vi "SignalConversion.vi"(1 "Method for Zbead calculation (hard coded)":u16(ring) items=["Linear", "Polynomial", "Lookup table"], 6 "Reinitialize time? (F)":bool, 8 "error in (no error)":errorcluster, 9 "All data after scaling":T2, 10 "All DAQ channels":T1, 11 "Params in":T8={"Manual Control"={"Rotation Control"={"Phase"=0.0, "A amp (0-120)"=75.0, "B amp (0-120)"=53.3, "mean freq  [MHz]\ndefault 39.99"=40.0, "freq difference [Hz]"=2.0, "Enable A"=TRUE, "Enable B"=TRUE}, "X piezo\n [nm]"=0.0, "Y peizo\n [nm]"=0.0, "-Z piezo\n [nm]"=5.012658227848101, "AOM0 \nPower"=0.2}, "Piezo Calibr"={"Px2Vx(AO)"=nan, "Py2Vy(AO)"=nan, "Pz2Vz(AO)"=nan, "Min Px"=nan, "Min Py"=nan, "Min Pz"=nan, "Max Px"=nan, "Max Py"=nan, "Max Pz"=nan, "Vx0 (V)"=nan, "Vy0 (V)"=nan, "Vz0 (V)"=nan}, "Instrument Calibr"={"Angular compensation coeffs"=[], "TetherCenter"={"TrapX_AO 0 [nm]"=nan, "TrapY_AO 0 [nm]"=nan, "TrapZ_AO 0 [nm]"=nan}, "XYZsignal baseline"={"Xsignal0"=nan, "Ysignal0"=nan, "Zsignal0"=nan, "Zsig slope"=nan, "Z bead0"=nan}, "S and P to Vs0"={"Vs0/P"=1.0, "Vs0/S"=1.0}, "Psi"=0.0, "ePS:eRL drift correlation"={"Interc P"=nan, "Slope P"=nan, "Interc S"=nan, "Slope S"=nan}, "Current piezo volt AO"={"Vpx_AO [V]"=nan, "Vpy_AO [V]"=nan, "Vpz_AO [V]"=nan}}, "Cylinder Calibr"={"ZStiff"=nan, "Zsens"=nan, "AngStiff"=nan, "XStiff"=nan, "Xsens"=nan, "MaxEllip"=nan, "YStiff"=nan, "Ysens"=nan, "FocalShift"=nan, "Sfz"=nan, "1/Sz"=nan, "Stau"=nan, "Sfx"=nan, "1/Sx"=nan, "1/Sang"=nan, "Sfy"=nan, "1/Sy"=nan, "1/focal"=nan}, "DAQParams"={"Buffer size"=nan, "Scanning rate"=nan, "Average"=nan, "Sampling rate"=nan, "set dt"=nan}, "DAQ channel offsets"={"A0 [V]"=0.0, "D0 [V]"=0.0, "P0  [V]"=0.0, "S0 [V]"=0.0, "L0 [V]"=0.0, "R0 [V]"=0.0, "Vpx0 [V]"=0.0, "Vpy0 [V]"=0.0, "Vpz0 [V]"=0.0, "Vsum0 [V]"=0.0, "Vpx_AO0 [V]"=0.0, "Vpy_AO0 [V]"=0.0, "Vpz_AO0 [V]"=0.0}, "Z bead polynomial coeffs"=[nan, nan, nan, nan], "Skip button ref"=refnum, "z bead lookup table"={"z signal"=[], "z bead"=[]}, "SP->power Matrix"=[], "Ms2p"=[], "Mp2s"=[], "Polynomial coeff V_px,y,z 2 position (nm)"=[], "task in"=""} {"Instrument Calibr"."Psi" format="%#_2f"; "Manual Control"."Y peizo\n [nm]" scale=0.0..7000.0; "Manual Control"."AOM0 \nPower" scale=0.0..1.0; "Manual Control"."X piezo\n [nm]" scale=0.0..7000.0; "Manual Control"."Rotation Control"."freq difference [Hz]" step=0.5; "Manual Control"."Rotation Control"."mean freq  [MHz]\ndefault 39.99" min=0.0 step=0.01; "Manual Control"."Rotation Control"."B amp (0-120)" min=0.0 max=120.0 step=0.1; "Manual Control"."Rotation Control"."A amp (0-120)" min=0.0 max=120.0 step=0.1; "Manual Control"."Rotation Control"."Phase" scale=0.0..360.0; "Manual Control"."-Z piezo\n [nm]" scale=1000.0..7000.0}) -> (0 "error out":errorcluster, 2 "Physical Quantities cluster out":T13, 3 "Params out":T8={"Manual Control"={"Rotation Control"={"Phase"=0.0, "A amp (0-120)"=75.0, "B amp (0-120)"=53.3, "mean freq  [MHz]\ndefault 39.99"=40.0, "freq difference [Hz]"=2.0, "Enable A"=TRUE, "Enable B"=TRUE}, "X piezo\n [nm]"=0.0, "Y peizo\n [nm]"=0.0, "-Z piezo\n [nm]"=5.012658227848101, "AOM0 \nPower"=0.2}, "Piezo Calibr"={"Px2Vx(AO)"=nan, "Py2Vy(AO)"=nan, "Pz2Vz(AO)"=nan, "Min Px"=nan, "Min Py"=nan, "Min Pz"=nan, "Max Px"=nan, "Max Py"=nan, "Max Pz"=nan, "Vx0 (V)"=nan, "Vy0 (V)"=nan, "Vz0 (V)"=nan}, "Instrument Calibr"={"Angular compensation coeffs"=[], "TetherCenter"={"TrapX_AO 0 [nm]"=nan, "TrapY_AO 0 [nm]"=nan, "TrapZ_AO 0 [nm]"=nan}, "XYZsignal baseline"={"Xsignal0"=nan, "Ysignal0"=nan, "Zsignal0"=nan, "Zsig slope"=nan, "Z bead0"=nan}, "S and P to Vs0"={"Vs0/P"=1.0, "Vs0/S"=1.0}, "Psi"=0.0, "ePS:eRL drift correlation"={"Interc P"=nan, "Slope P"=nan, "Interc S"=nan, "Slope S"=nan}, "Current piezo volt AO"={"Vpx_AO [V]"=nan, "Vpy_AO [V]"=nan, "Vpz_AO [V]"=nan}}, "Cylinder Calibr"={"ZStiff"=nan, "Zsens"=nan, "AngStiff"=nan, "XStiff"=nan, "Xsens"=nan, "MaxEllip"=nan, "YStiff"=nan, "Ysens"=nan, "FocalShift"=nan, "Sfz"=nan, "1/Sz"=nan, "Stau"=nan, "Sfx"=nan, "1/Sx"=nan, "1/Sang"=nan, "Sfy"=nan, "1/Sy"=nan, "1/focal"=nan}, "DAQParams"={"Buffer size"=nan, "Scanning rate"=nan, "Average"=nan, "Sampling rate"=nan, "set dt"=nan}, "DAQ channel offsets"={"A0 [V]"=0.0, "D0 [V]"=0.0, "P0  [V]"=0.0, "S0 [V]"=0.0, "L0 [V]"=0.0, "R0 [V]"=0.0, "Vpx0 [V]"=0.0, "Vpy0 [V]"=0.0, "Vpz0 [V]"=0.0, "Vsum0 [V]"=0.0, "Vpx_AO0 [V]"=0.0, "Vpy_AO0 [V]"=0.0, "Vpz_AO0 [V]"=0.0}, "Z bead polynomial coeffs"=[nan, nan, nan, nan], "Skip button ref"=refnum, "z bead lookup table"={"z signal"=[], "z bead"=[]}, "SP->power Matrix"=[], "Ms2p"=[], "Mp2s"=[], "Polynomial coeff V_px,y,z 2 position (nm)"=[], "task in"=""} {"Instrument Calibr"."Psi" format="%#_2f"; "Manual Control"."Y peizo\n [nm]" scale=0.0..7000.0; "Manual Control"."AOM0 \nPower" scale=0.0..1.0; "Manual Control"."X piezo\n [nm]" scale=0.0..7000.0; "Manual Control"."Rotation Control"."freq difference [Hz]" step=0.5; "Manual Control"."Rotation Control"."mean freq  [MHz]\ndefault 39.99" min=0.0 step=0.01; "Manual Control"."Rotation Control"."B amp (0-120)" min=0.0 max=120.0 step=0.1; "Manual Control"."Rotation Control"."A amp (0-120)" min=0.0 max=120.0 step=0.1; "Manual Control"."Rotation Control"."Phase" scale=0.0..360.0; "Manual Control"."-Z piezo\n [nm]" scale=1000.0..7000.0})   [LabVIEW 2017, in "SignalConverson.lvlib"]
uses:
  SignalConverson.lvlib
  Initialization/New Param_170907.ctl
  Initialization/ManualCtrl.ctl
  Initialization/CylinderCalibrNew.ctl
  DAQChannelOffsets.ctl
  <vilib>/Analysis/Matrix/Datatypes/RealMatrix.ctl
  Initialization/Physical Quantitites.ctl
  ScaledData.ctl
  Measrured TrapXYZ.ctl
  Data Before Angle Compensation.ctl
  Angle compensated data.ctl
  XYZ Signals.ctl
  Set TrapXYZ.ctl
  DAQChannelRawData.ctl
  <vilib>/Analysis/polynomials.llb/Scalar Polynomial Evaluation (DBL).vi
  <vilib>/Analysis/NI_AALPro.lvlib
  Initialization/Initialization.lvlib
  <vilib>/Analysis/Matrix/NI_Matrix.lvlib
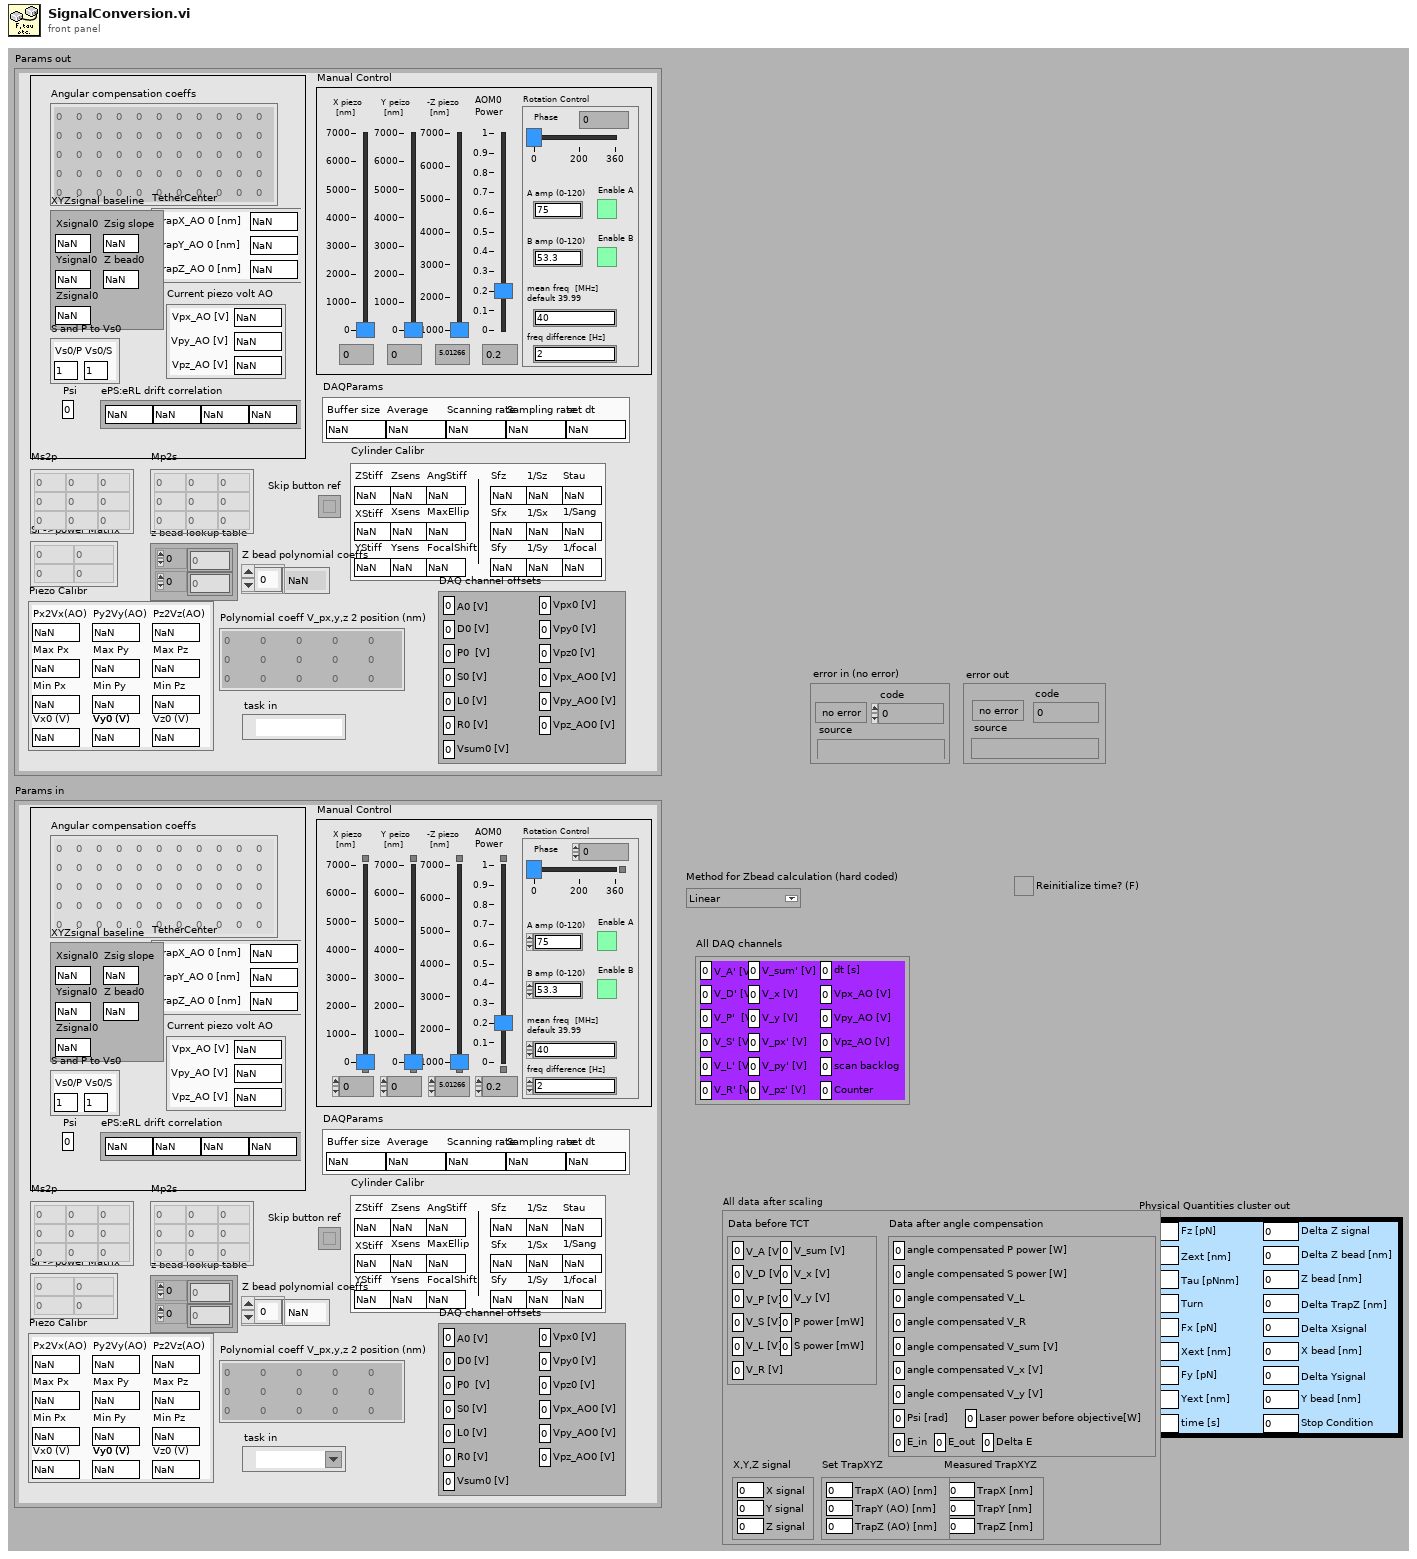
[diagram p1: front panel]
types:
  T1 = typedef "SignalConverson.lvlib/DAQChannelRawData.ctl" = cluster{"V_A' [V]":dbl, "V_D' [V]":dbl, "V_P'  [V]":dbl, "V_S' [V]":dbl, "V_L' [V]":dbl, "V_R' [V]":dbl, "V_sum' [V]":dbl, "V_x [V]":dbl, "V_y [V]":dbl, "V_px' [V]":dbl, "V_py' [V]":dbl, "V_pz' [V]":dbl, "dt [s]":dbl, "Vpx_AO [V]":dbl, "Vpy_AO [V]":dbl, "Vpz_AO [V]":dbl, "scan backlog":u32, "Counter":u32}
  T2 = typedef "SignalConverson.lvlib/ScaledData.ctl" = cluster{"Measured TrapXYZ":T3, "Data before TCT":T4, "Data after angle compensation":T5, "X,Y,Z signal":T6, "Set TrapXYZ":T7}
  T3 = typedef "SignalConverson.lvlib/Measrured TrapXYZ.ctl" = cluster{"TrapX [nm]":dbl, "TrapY [nm]":dbl, "TrapZ [nm]":dbl}
  T4 = typedef "SignalConverson.lvlib/Data Before Angle Compensation.ctl" = cluster{"V_A [V]":dbl, "V_D [V]":dbl, "V_P [V]":dbl, "V_S [V]":dbl, "V_L [V]":dbl, "V_R [V]":dbl, "V_sum [V]":dbl, "V_x [V]":dbl, "V_y [V]":dbl, "P power [mW]":dbl, "S power [mW]":dbl}
  T5 = typedef "SignalConverson.lvlib/Angle compensated data.ctl" = cluster{"angle compensated P power [W]":dbl, "angle compensated S power [W]":dbl, "angle compensated V_L":dbl, "angle compensated V_R":dbl, "angle compensated V_sum [V]":dbl, "angle compensated V_x [V]":dbl, "angle compensated V_y [V]":dbl, "Psi [rad]":dbl, "Laser power before objective[W]":dbl, "E_in":dbl, "E_out":dbl, "Delta E":dbl}
  T6 = typedef "SignalConverson.lvlib/XYZ Signals.ctl" = cluster{"X signal":dbl, "Y signal":dbl, "Z signal":dbl}
  T7 = typedef "SignalConverson.lvlib/Set TrapXYZ.ctl" = cluster{"TrapX (AO) [nm]":dbl, "TrapY (AO) [nm]":dbl, "TrapZ (AO) [nm]":dbl}
  T8 = typedef "Initialization.lvlib/New Param_170907.ctl" = cluster{"Manual Control":T9, "Piezo Calibr":cluster{"Px2Vx(AO)":dbl, "Py2Vy(AO)":dbl, "Pz2Vz(AO)":dbl, "Min Px":dbl, "Min Py":dbl, "Min Pz":dbl, "Max Px":dbl, "Max Py":dbl, "Max Pz":dbl, "Vx0 (V)":dbl, "Vy0 (V)":dbl, "Vz0 (V)":dbl}, "Instrument Calibr":cluster{"Angular compensation coeffs":dbl[][], "TetherCenter":cluster{"TrapX_AO 0 [nm]":dbl, "TrapY_AO 0 [nm]":dbl, "TrapZ_AO 0 [nm]":dbl}, "XYZsignal baseline":cluster{"Xsignal0":dbl, "Ysignal0":dbl, "Zsignal0":dbl, "Zsig slope":dbl, "Z bead0":dbl}, "S and P to Vs0":cluster{"Vs0/P":dbl, "Vs0/S":dbl}, "Psi":dbl, "ePS:eRL drift correlation":cluster{"Interc P":dbl, "Slope P":dbl, "Interc S":dbl, "Slope S":dbl}, "Current piezo volt AO":cluster{"Vpx_AO [V]":dbl, "Vpy_AO [V]":dbl, "Vpz_AO [V]":dbl}}, "Cylinder Calibr":T10, "DAQParams":cluster{"Buffer size":dbl, "Scanning rate":dbl, "Average":dbl, "Sampling rate":dbl, "set dt":dbl}, "DAQ channel offsets":T11, "Z bead polynomial coeffs":dbl[], "Skip button ref":refnum<vi>, "z bead lookup table":cluster{"z signal":dbl[], "z bead":dbl[]}, "SP->power Matrix":T12, "Ms2p":T12, "Mp2s":T12, "Polynomial coeff V_px,y,z 2 position (nm)":dbl[][], "task in":refnum<k21>}
  T9 = typedef "Initialization.lvlib/ManualCtrl.ctl" = cluster{"Rotation Control":cluster{"Phase":dbl, "A amp (0-120)":dbl, "B amp (0-120)":dbl, "mean freq  [MHz]\ndefault 39.99":dbl, "freq difference [Hz]":dbl, "Enable A":bool, "Enable B":bool}, "X piezo\n [nm]":dbl, "Y peizo\n [nm]":dbl, "-Z piezo\n [nm]":dbl, "AOM0 \nPower":dbl}
  T10 = typedef "Initialization.lvlib/CylinderCalibrNew.ctl" = cluster{"ZStiff":dbl, "Zsens":dbl, "AngStiff":dbl, "XStiff":dbl, "Xsens":dbl, "MaxEllip":dbl, "YStiff":dbl, "Ysens":dbl, "FocalShift":dbl, "Sfz":dbl, "1/Sz":dbl, "Stau":dbl, "Sfx":dbl, "1/Sx":dbl, "1/Sang":dbl, "Sfy":dbl, "1/Sy":dbl, "1/focal":dbl}
  T11 = typedef "SignalConverson.lvlib/DAQChannelOffsets.ctl" = cluster{"A0 [V]":dbl, "D0 [V]":dbl, "P0  [V]":dbl, "S0 [V]":dbl, "L0 [V]":dbl, "R0 [V]":dbl, "Vpx0 [V]":dbl, "Vpy0 [V]":dbl, "Vpz0 [V]":dbl, "Vsum0 [V]":dbl, "Vpx_AO0 [V]":dbl, "Vpy_AO0 [V]":dbl, "Vpz_AO0 [V]":dbl}
  T12 = typedef "NI_Matrix.lvlib/RealMatrix.ctl" = dbl[][]
  T13 = typedef "SignalConverson.lvlib/Physical Quantitites.ctl" = cluster{"Fz [pN]":dbl, "Zext [nm]":dbl, "Tau [pNnm]":dbl, "Turn":dbl, "Fx [pN]":dbl, "Xext [nm]":dbl, "Fy [pN]":dbl, "Yext [nm]":dbl, "time [s]":dbl, "Delta Z signal":dbl, "Delta Z bead [nm]":dbl, "Z bead [nm]":dbl, "Delta TrapZ [nm]":dbl, "Delta Xsignal":dbl, "X bead [nm]":dbl, "Delta Ysignal":dbl, "Y bead [nm]":dbl, "Stop Condition":dbl}
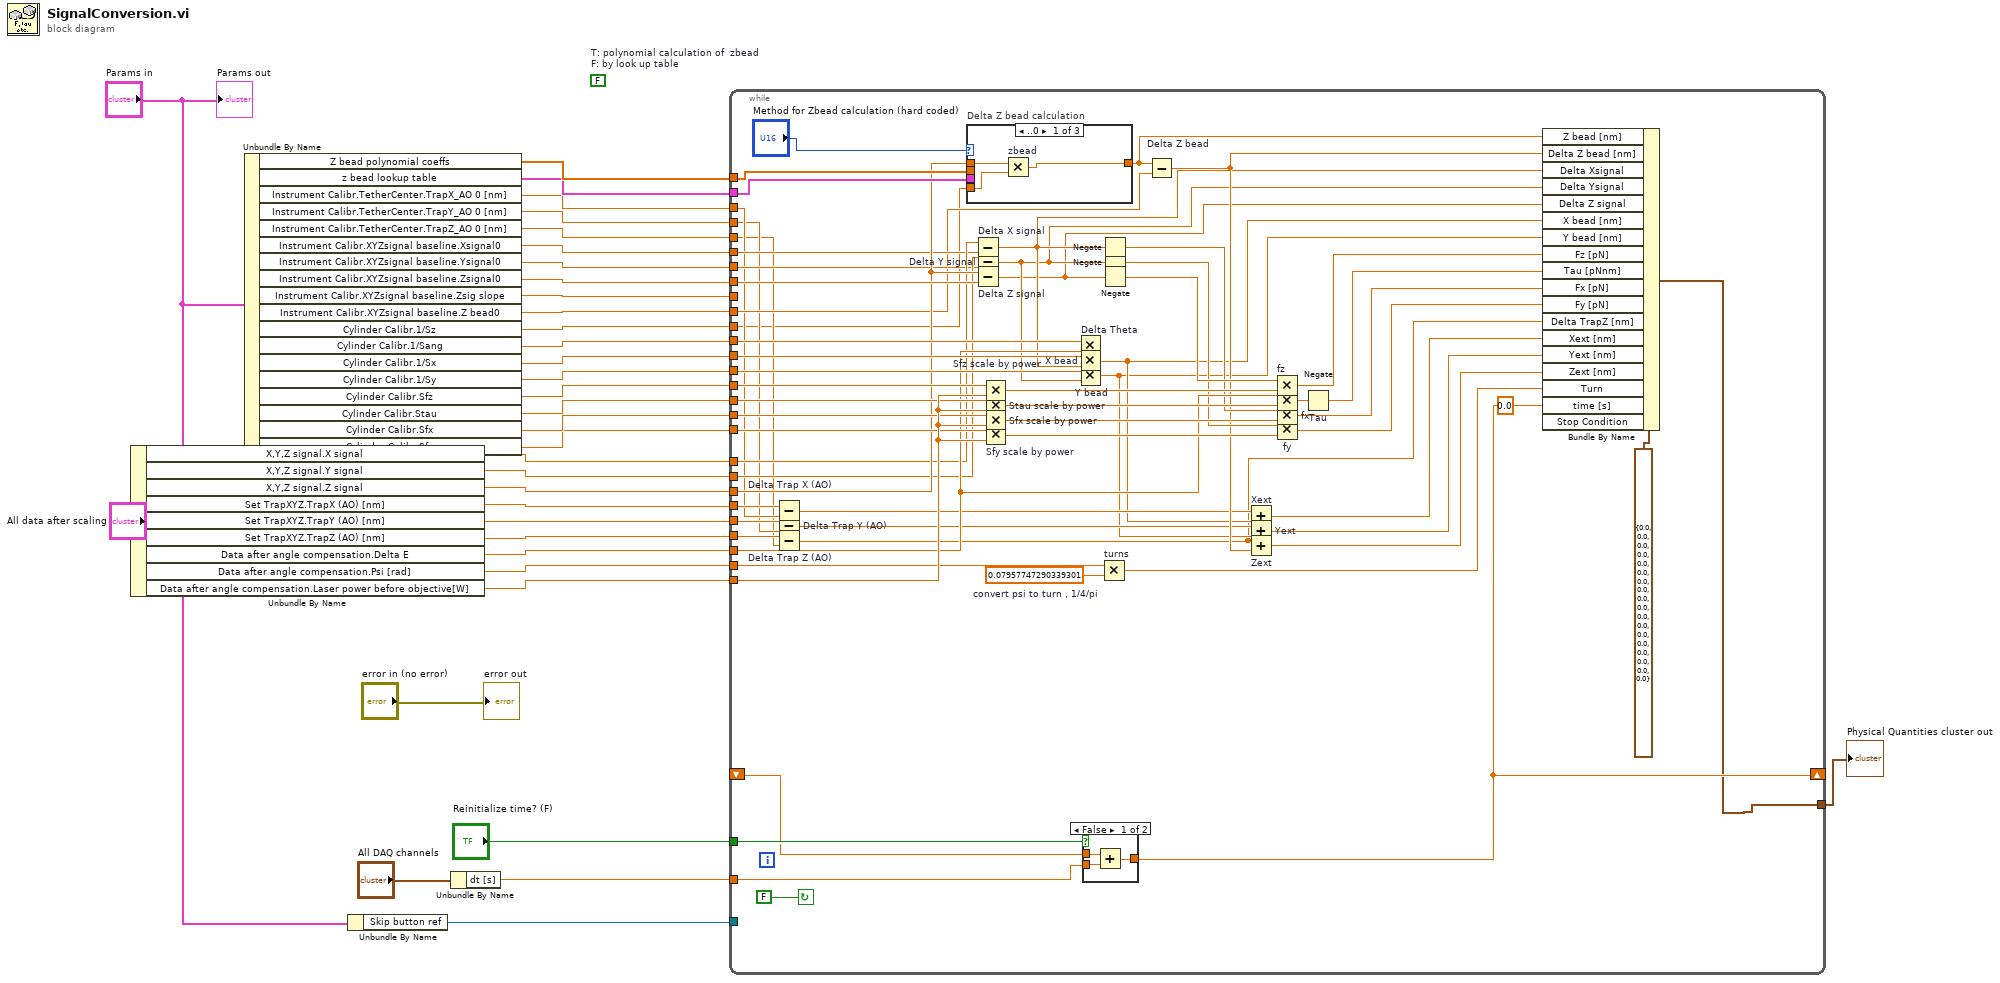
[diagram p0: block diagram]
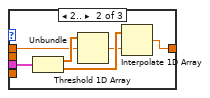
[diagram p2: hidden frame]
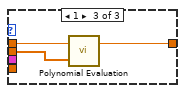
[diagram p3: hidden frame]
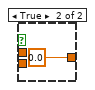
[diagram p4: hidden frame]
diagram:
  (unwired) FALSE  # T: polynomial calculation of  zbead F: by look up table
  n1 = Unbundle By Name("All data after scaling") -> ("X,Y,Z signal.X signal"=w29:dbl, "X,Y,Z signal.Y signal"=w30:dbl, "X,Y,Z signal.Z signal"=w31:dbl, "Set TrapXYZ.TrapX (AO) [nm]"=w28:dbl, "Set TrapXYZ.TrapY (AO) [nm]"=w27:dbl, "Set TrapXYZ.TrapZ (AO) [nm]"=w26:dbl, "Data after angle compensation.Delta E"=w25:dbl, "Data after angle compensation.Psi [rad]"=w24:dbl, "Data after angle compensation.Laser power before objective[W]"=w21:dbl)
  n2 = Unbundle By Name("Params in") -> ("Z bead polynomial coeffs"=w34:dbl[], "z bead lookup table"=w33:cluster{"z signal":dbl[], "z bead":dbl[]}, "Instrument Calibr.TetherCenter.TrapX_AO 0 [nm]"=w20:dbl, "Instrument Calibr.TetherCenter.TrapY_AO 0 [nm]"=w19:dbl, "Instrument Calibr.TetherCenter.TrapZ_AO 0 [nm]"=w18:dbl, "Instrument Calibr.XYZsignal baseline.Xsignal0"=w17:dbl, "Instrument Calibr.XYZsignal baseline.Ysignal0"=w16:dbl, "Instrument Calibr.XYZsignal baseline.Zsignal0"=w15:dbl, "Instrument Calibr.XYZsignal baseline.Zsig slope"=w14:dbl, "Instrument Calibr.XYZsignal baseline.Z bead0"=w13:dbl, "Cylinder Calibr.1/Sz"=w12:dbl, "Cylinder Calibr.1/Sang"=w11:dbl, "Cylinder Calibr.1/Sx"=w10:dbl, "Cylinder Calibr.1/Sy"=w9:dbl, "Cylinder Calibr.Sfz"=w8:dbl, "Cylinder Calibr.Stau"=w7:dbl, "Cylinder Calibr.Sfx"=w6:dbl, "Cylinder Calibr.Sfy"=w5:dbl)
  n3 = Unbundle By Name("Params in") -> ("Skip button ref"=w4:refnum<vi>)
  n4 = Unbundle By Name("All DAQ channels") -> ("dt [s]"=w22:dbl)
  n5 = while {
    tunnel: "Reinitialize time? (F)" -> [w96]
    shift-right: [w46] -> _
    shift-left: _ -> [w95]
    tunnel: w34 -> [w93]
    tunnel: w33 -> [w94]
    tunnel: w31 -> [w81]
    tunnel: w30 -> [w74]
    tunnel: w29 -> [w73]
    tunnel: w28 -> [w63]
    tunnel: w27 -> [w62]
    tunnel: w26 -> [w61]
    tunnel: w25 -> [w75]
    tunnel: w24 -> [w69]
    tunnel: w22 -> [w89]
    tunnel: w21 -> [w92]
    tunnel: w20 -> [w60]
    tunnel: w19 -> [w59]
    tunnel: w18 -> [w58]
    tunnel: w17 -> [w71]
    tunnel: w16 -> [w72]
    tunnel: w15 -> [w91]
    tunnel: w14 -> [_]
    tunnel: w13 -> [w66]
    tunnel: w12 -> [w39]
    tunnel: w11 -> [w84]
    tunnel: w10 -> [w83]
    tunnel: w9 -> [w82]
    tunnel: w8 -> [w85]
    tunnel: w7 -> [w86]
    tunnel: w6 -> [w87]
    tunnel: w5 -> [w88]
    tunnel: w4 -> [_]
    tunnel: [w36] -> w2
    stop <- FALSE continue-if-true
    w70 = 0.07957747290339301  # convert psi to turn , 1/4/pi
    n6 = Subtract "Delta Trap X (AO)"(x=w63, y=w60) -> (x-y=w57:dbl)
    n7 = Subtract "Delta Trap Y (AO)"(x=w62, y=w59) -> (x-y=w56:dbl)
    n8 = Subtract "Delta Trap Z (AO)"(x=w61, y=w58) -> (x-y=w44:dbl)
    n9 = case "Delta Z bead calculation" shown="..0" "Method for Zbead calculation (hard coded)" {
      tunnel: w93 -> [_ _ w109]
      tunnel: w81 -> [w100 w104 w108]
      tunnel: [w98 w101 w107] -> w65
      tunnel: w94 -> [_ w106 _]
      tunnel: w39 -> [w99 _ _]
      frame ..0 {
        n10 = Multiply "zbead"(x=w100, y=w99) -> (x*y=w98:dbl)
      }
      frame 2.. {
        n11 = Unbundle(w106) -> ("z signal"=w105:dbl[], "z bead"=w103:dbl[])
        n12 = Threshold 1D Array(2:w104, 3:w105) -> (0:w102:dbl)  [unwired: 1 in]
        n13 = Interpolate 1D Array(1:w102, 2:w103) -> (0:w101:dbl)
      }
      frame 1 {
        n14 = call-poly <vilib>:"Polynomial Evaluation.vi"("P(x)"=w109, "a"=w108) -> ("P(a)"=w107:dbl)  [unwired: 1 out]
      }
    }
    n15 = Subtract "Delta X signal"(x=w73, y=w71) -> (x-y=w55:dbl)
    n16 = Subtract "Delta Y signal"(x=w74, y=w72) -> (x-y=w54:dbl)
    n17 = Subtract "Delta Z signal"(x=w81, y=w91) -> (x-y=w53:dbl)
    n18 = Multiply "Sfz scale by power"(x=w85, y=w92) -> (x*y=w80:dbl)
    n19 = Multiply "Stau scale by power"(x=w86, y=w92) -> (x*y=w79:dbl)
    n20 = Multiply "Sfx scale by power"(x=w87, y=w92) -> (x*y=w78:dbl)
    n21 = Multiply "Sfy scale by power"(x=w88, y=w92) -> (x*y=w77:dbl)
    n22 = Multiply "Delta Theta"(x=w84, y=w75) -> ()  [unwired: 1 out]
    n23 = Multiply "X bead"(x=w83, y=w55) -> (x*y=w49:dbl)
    n24 = Multiply "Y bead"(x=w82, y=w54) -> (x*y=w48:dbl)
    n25 = case shown="False" w96 {
      tunnel: w95 -> [w111 _]
      tunnel: [w112 0.0] -> w46
      tunnel: w89 -> [w110 _]
      frame False {
        n26 = Add(x=w111, y=w110) -> (x+y=w112:dbl)
      }
      frame True {
      }
    }
    n27 = Multiply "turns"(x=w69, y=w70) -> (x*y=w45:dbl)
    n28 = Negate ("The direction of force and Z signal are opposite")(x=w55) -> (-x=w67:dbl)
    n29 = Negate ("The direction of force and Z signal are opposite")(x=w54) -> (-x=w68:dbl)
    n30 = Negate ("The direction of force and Z signal are opposite")(x=w53) -> (-x=w76:dbl)
    n31 = Subtract "Delta Z bead"(x=w65, y=w66) -> (x-y=w64:dbl)
    n32 = Add "Xext"(x=w57, y=w49) -> (x+y=w43:dbl)
    n33 = Add "Yext"(x=w56, y=w48) -> (x+y=w41:dbl)
    n34 = Add "Zext"(x=w44, y=w64) -> (x+y=w42:dbl)
    n35 = Multiply "fz"(x=w76, y=w80) -> (x*y=w52:dbl)
    n36 = Multiply(x=w75, y=w79) -> (x*y=w38:dbl)
    n37 = Multiply "fx"(x=w67, y=w78) -> (x*y=w51:dbl)
    n38 = Multiply "fy"(x=w68, y=w77) -> (x*y=w50:dbl)
    n39 = Negate "Tau"(x=w38) -> (-x=w37:dbl)
    n40 = Bundle By Name(cluster=T13 {"Fz [pN]"=0.0, "Zext [nm]"=0.0, "Tau [pNnm]"=0.0, "Turn"=0.0, "Fx [pN]"=0.0, "Xext [nm]"=0.0, "Fy [pN]"=0.0, "Yext [nm]"=0.0, "time [s]"=0.0, "Delta Z signal"=0.0, "Delta Z bead [nm]"=0.0, "Z bead [nm]"=0.0, "Delta TrapZ [nm]"=0.0, "Delta Xsignal"=0.0, "X bead [nm]"=0.0, "Delta Ysignal"=0.0, "Y bead [nm]"=0.0, "Stop Condition"=0.0} ("Physical Quantities cluster out"), "Z bead [nm]"=w65, "Delta Z bead [nm]"=w64, "Delta Xsignal"=w55, "Delta Ysignal"=w54, "Delta Z signal"=w53, "X bead [nm]"=w49, "Y bead [nm]"=w48, "Fz [pN]"=w52, "Tau [pNnm]"=w37, "Fx [pN]"=w51, "Fy [pN]"=w50, "Delta TrapZ [nm]"=w44, "Xext [nm]"=w43, "Yext [nm]"=w41, "Zext [nm]"=w42, "Turn"=w45, "time [s]"=w46, "Stop Condition"=0.0) -> (w36:T13)
  }
  "Physical Quantities cluster out" <- w2
  "Params out" <- "Params in"
  "error out" <- "error in (no error)"
